vi "UsrProfiles-Compare user profile.vi"(8 "error in":errorcluster, 11 "Which profile?":T1) -> (0 "error out":errorcluster, 3 "Changes exist":bool)   [LabVIEW 2017]
uses:
  Typedefs/Which path.ctl
  Typedefs/Save-Load enum.ctl
  Typedefs/HW config states enum.ctl
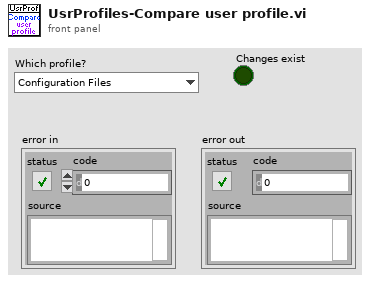
[diagram p1: front panel]
types:
  T1 = typedef "Which path.ctl" = enum16{"Configuration Files", "Calibration Files", "Images", "Setup.ini", "Loaded User profile.ini", "User's-Previous session.ini", "New user profile.ini", "Selected User profile.ini", "User profiles folder", "Power meter scaling.txt", "FOV Cal.ini", "Calibration.ini"}
  T2 = typedef "HW config states enum.ctl" = enum16{"Load from file", "Save to file", "Write all", "Read all", "Write XY stage settings", "Write DAQ FPGA settings", "Write Control FPGA settings", "Write Phys Channels", "Clear", "Compare from file"}
  T3 = typedef "Save-Load enum.ctl" = enum16{"Save to file", "Load from file", "Compare from file"}
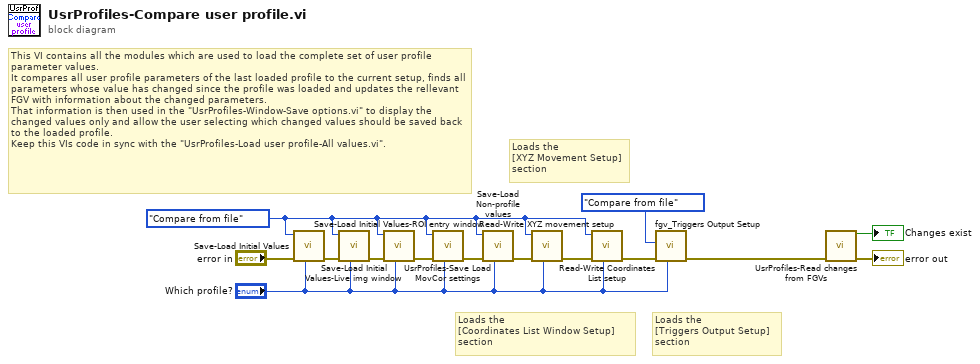
[diagram p0: block diagram]
diagram:
  w2 = Save-Load_enum."Compare from file" ("Function")
  # "Loads the\n[Triggers Output Setup]\nsection"
  # "Loads the\n[Coordinates List Window Setup]\nsection"
  # "Loads the\n[XYZ Movement Setup]\nsection"
  # "This VI contains all the modules which are used to load the complete set of user profile parameter values.\nIt compares all user profile parameters of the last loaded profile to the current setup, finds all parameters whose value has changed since the profile was loaded and updates the rellevant FGV with information about the changed parameters.\nThat information is then used in the \"UsrProfiles-Window-Save options.vi\" to display the changed values only and allow the user selecting which changed values should be saved back to the loaded profile.\nKeep this VIs code in sync with the \"UsrProfiles-Load user profile-All values.vi\"."
  n1 = call "Save-Load Initial Values.vi"("Which file? (User profile.ini)"="Which profile?", "error in"="error in", "Function"=w2) -> ("error out"=w12:errorcluster)  [unwired: 8 in]
  n2 = call "Save-Load Initial Values-Live img window.vi"("Which file? (User profile.ini)"="Which profile?", "error in"=w12, "Function"=w2) -> ("error out"=w13:errorcluster)  [unwired: 8 in]
  n3 = call "Save-Load Initial Values-ROI entry window.vi"("Which file? (User profile.ini)"="Which profile?", "error in"=w13, "Function"=w2) -> ("error out"=w14:errorcluster)  [unwired: 8 in]
  n4 = call "UsrProfiles-Save Load MovCor settings.vi"("Which file? (User profile.ini)"="Which profile?", "error in (no error)"=w14, "Function"=w2) -> ("error out"=w10:errorcluster)  [unwired: 8 in]
  n5 = call "Save-Load Non-profile values.vi"("Which file? (User profile.ini)"="Which profile?", "error in"=w10, "Function"=w2) -> ("error out"=w4:errorcluster)  [unwired: 8 in]
  n6 = call "Read-Write XYZ movement setup.vi"("Which file? (User profile.ini)"="Which profile?", "error in"=w4, "Function"=w2) -> ("error out"=w7:errorcluster)  [unwired: 8 in]
  n7 = call "Read-Write Coordinates List setup.vi"("Which file?"="Which profile?", "error in"=w7, "Function"=w2) -> ("error out"=w6:errorcluster)  [unwired: 8 in]
  n8 = call "fgv_Triggers Output Setup.vi"("Which file? (User profile.ini)"="Which profile?", "error in (no error)"=w6, "Function"=HW_config_states_enum."Compare from file") -> ("error out"=w3:errorcluster)  [unwired: 6 in, 2 out]
  n9 = call "UsrProfiles-Read changes from FGVs.vi"("error in (no error)"=w3) -> ("Changes exist"=→"Changes exist":bool, "error out"=→"error out":errorcluster)  [unwired: 9 in, 4 out]
